vi "Joystick RefNum.vi"() -> ()   [LabVIEW 2018]
panel:
  in  "Legal_Drivers":string[](array[string])=["Ethan", "Adam", "Amelia"]
  out "Joystick_1":string
  out "Joystick_0":string
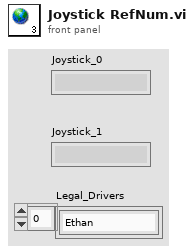
[diagram p1: front panel]
diagram:
